vi "Delete Polymorphic.vi"   [LabVIEW 2020, in "NI_VIAnCFGDataStructure.lvlib" / "Tree.lvclass"]
doc: "Polymorphic instance of the Delete method. Select the appropraite instance to work with or allow this method to adapt automatically."
uses:
  <vilib>/addons/analyzer/VIAnCFGDataStructure/Tree Manager/Tree.lvclass
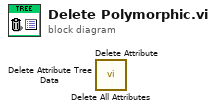
[diagram p0: block diagram]
diagram:
  n1 = call <vilib>:"Delete All Attributes.vi"() -> ()  [unwired: 10 in, 2 out]
  n2 = call <vilib>:"Delete Attribute.vi"() -> ()  [unwired: 8 in, 4 out]
  n3 = call <vilib>:"Delete Attribute Tree Data.vi"() -> ()  [unwired: 8 in, 4 out]
